vi "Populate Objects Lists.vi"(8 "error in":errorcluster, 11 "UI Actor in":refnum<class "UI Actor.lvclass">) -> (0 "error out":errorcluster, 3 "UI Actor out":refnum<class "UI Actor.lvclass">)   [LabVIEW 2024, in "UI Actor.lvlib" / "UI Actor.lvclass"]
uses:
  UI Actor.lvclass
  UI Actor.lvclass/UI Actor.ctl
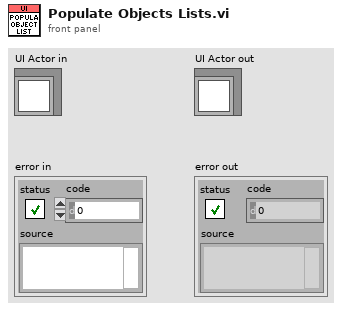
[diagram p1: front panel]
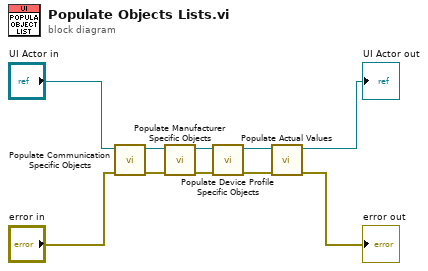
[diagram p0: block diagram]
diagram:
  n1 = call "Populate Communication Specific Objects.vi"("error in"="error in", "UI Actor in"="UI Actor in") -> ("error out"=w8:errorcluster, "UI Actor out"=w6:refnum<class "UI Actor.lvclass">)  [unwired: 8 in]
  n2 = call "Populate Manufacturer Specific Objects.vi"("error in"=w8, "UI Actor in"=w6) -> ("error out"=w7:errorcluster, "UI Actor out"=w4:refnum<class "UI Actor.lvclass">)  [unwired: 8 in]
  n3 = call "Populate Device Profile Specific Objects.vi"("error in"=w7, "UI Actor in"=w4) -> ("error out"=w5:errorcluster, "UI Actor out"=w2:refnum<class "UI Actor.lvclass">)  [unwired: 8 in]
  n4 = call-dynamic "Populate Actual Values.vi"("error in"=w5, "UI Actor in"=w2) -> ("error out"=→"error out":errorcluster, "UI Actor out"=→"UI Actor out":refnum<class "UI Actor.lvclass">)  [unwired: 8 in]
